vi "VIs.vi"(1 "VI In":T1, 2 "Name":string) -> (0 "VI Out":T1)   [LabVIEW 2014]
uses:
  LabVIEW.vi
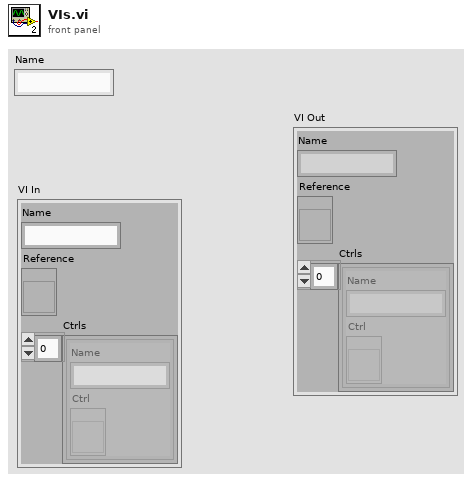
[diagram p1: front panel]
types:
  T1 = cluster{"Name":string, "Reference":refnum<vi>, "Ctrls":cluster{"Name":string, "Ctrl":refnum<vi>}[]}
  T2 = cluster{"Name":string, "Reference":refnum<vi>, "Ctrls":cluster{"Name":string, "Ctrl":refnum<vi>}[]}[]
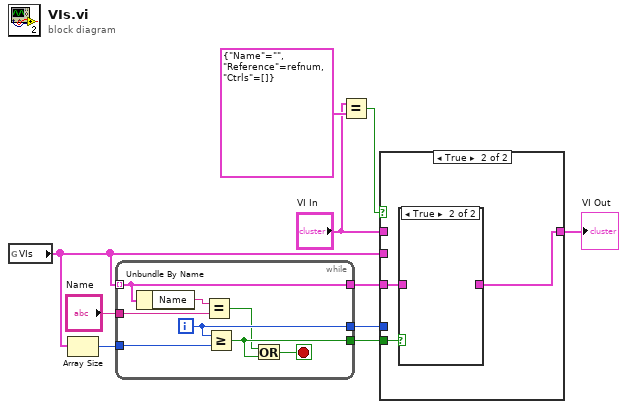
[diagram p0: block diagram]
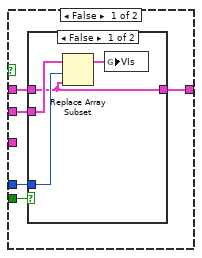
[diagram p2: hidden frame]
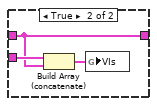
[diagram p3: hidden frame]
diagram:
  n1 = global read "LabVIEW.vi" "VIs"() -> (w1:T2)
  n2 = Array Size(array=w1) -> (size(s)=w3:i32)
  n3 = while {
    tunnel: w1 -> [w16] mode=indexing
    tunnel: "Name" -> [w17]
    tunnel: [w14] -> w5
    tunnel: [w16] -> w7
    tunnel: w3 -> [w15]
    tunnel: [w13] -> w2
    i -> [w14]
    stop <- w11 stop-if-true
    n4 = Unbundle By Name(w16) -> ("Name"=w18:string)
    n5 = Equal?(x=w18, y=w17) -> (x = y?=w12:bool)
    n6 = Greater Or Equal?(x=w14, y=w15) -> (x >= y?=w13:bool)
    n7 = Or(x=w12, y=w13) -> (x .or. y?=w11:bool)
  }
  n8 = Equal?(x="VI In", y=T1 {"Name"="", "Reference"=refnum, "Ctrls"=[]} ("VI In")) -> (x = y?=w8:bool)
  n9 = case shown="True" w8 {
    tunnel: w2 -> [w19 w33]
    tunnel: w7 -> [_ w32]
    tunnel: [w20 w31] -> w6
    tunnel: w1 -> [w23 _]
    tunnel: w5 -> [w22 _]
    tunnel: "VI In" -> [w21 _]
    frame False {
      n10 = case shown="False" w19 {
        tunnel: w23 -> [w27 w30]
        tunnel: w22 -> [w26 _]
        tunnel: w21 -> [w24 w28]
        tunnel: [w24 w28] -> w20
        frame False {
          n11 = Replace Array Subset(array=w27, new element=w24, index=w26) -> (w25:T2)
          n12 = global write "RemoteVIs.vi" "VIs"(w25) -> ()
        }
        frame True {
          n13 = Build Array (concatenate)(w30, w28) -> (w29:T2)
          n14 = global write "RemoteVIs.vi" "VIs"(w29) -> ()
        }
      }
    }
    frame True {
      n15 = case shown="True" w33 {
        tunnel: w32 -> [w34 _]
        tunnel: [w34 _] -> w31
        frame False {
        }
        frame True {
        }
      }
    }
  }
  "VI Out" <- w6
